vi "Remove Connected Client.vi"(8 "error in (no error)":errorcluster, 10 "GUID":string, 11 "Websocket Server in":refnum<class "WS Server.lvclass">) -> (0 "error out":errorcluster, 3 "Websocket Server out":refnum<class "WS Server.lvclass">)   [LabVIEW 2016, in "WebSocket Networking.lvlib" / "WS Server.lvclass"]
uses:
  <userlib>/Common Components/WebSocket Networking/WS Server/WS Server.lvclass
  C:/Program Files (x86)/National Instruments/LabVIEW 2016/user.lib/Composed Systems/Stream/Mediator/Classes/Websocket Server Actor/Websocket Server/Websocket Server.lvclass
  <userlib>/Common Components/WebSocket Networking/WS Server/WS Server.lvclass/WS Server.ctl
  <userlib>/Composed Systems/Stream/Mediator/Classes/Websocket Server Actor/Websocket Server/Websocket Server.lvclass
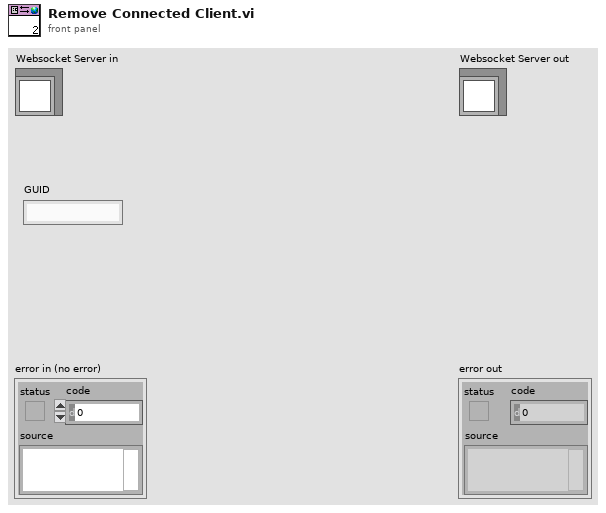
[diagram p1: front panel]
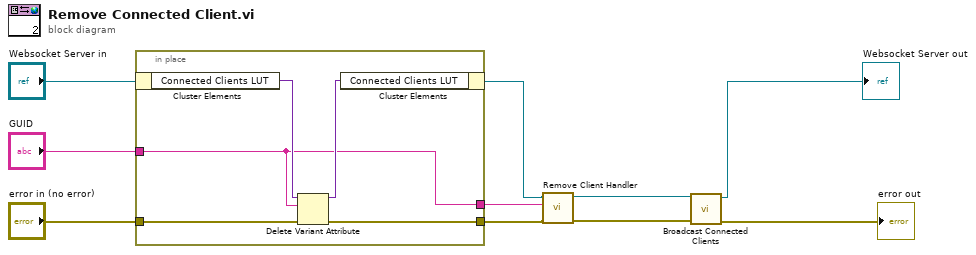
[diagram p0: block diagram]
diagram:
  n1 = in-place {
    in-place-border: "GUID" -> [w11]
    in-place-border: "error in (no error)" -> [w13]
    in-place-border: [w12] -> w3
    in-place-border: [w11] -> w1
    n2 = in-place-cluster #1("Websocket Server in") -> ("Connected Clients LUT"=w15:variant)
    n3 = Delete Variant Attribute(4:w13, 6:w11, 7:w15) -> (0:w12:errorcluster, 3:w14:variant)  [unwired: 1 out]
    n4 = in-place-cluster #1("Connected Clients LUT"=w14) -> (w5:refnum<class "WS Server.lvclass">)
  }
  n5 = call <userlib>:"Remove Client Handler.vi"("error in (no error)"=w3, "GUID"=w1, "Websocket Server in"=w5) -> ("error out"=w2:errorcluster, "Websocket Server out"=w4:refnum<class "WS Server.lvclass">)  [unwired: 7 in]
  n6 = call <userlib>:"Broadcast Connected Clients.vi"("error in (no error)"=w2, "Websocket Server in"=w4) -> ("error out"=→"error out":errorcluster, "Websocket Server out"=→"Websocket Server out":refnum<class "WS Server.lvclass">)  [unwired: 8 in]
